vi "Find Multiple by Path Test.vi"() -> ()   [LabVIEW 2017]
uses:
  String Subset.vi
  support/Strip Quotes and Unescape.vi
  Parsing/Parse Full Path or Item Name.vi
  Offset/Find Item Locations by Path.vi
  support/Unescape JSON string.vi
  support/Format JSON Object.vi
  <vilib>/addons/_JKI Toolkits/Caraya/classes/Test/Test.lvclass
  <vilib>/addons/_JKI Toolkits/Caraya/classes/Assert/Assert.lvclass
  JSONtext.lvlib
panel:
  out "Array":string[](array[string])
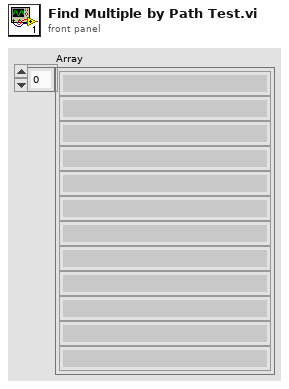
[diagram p1: front panel]
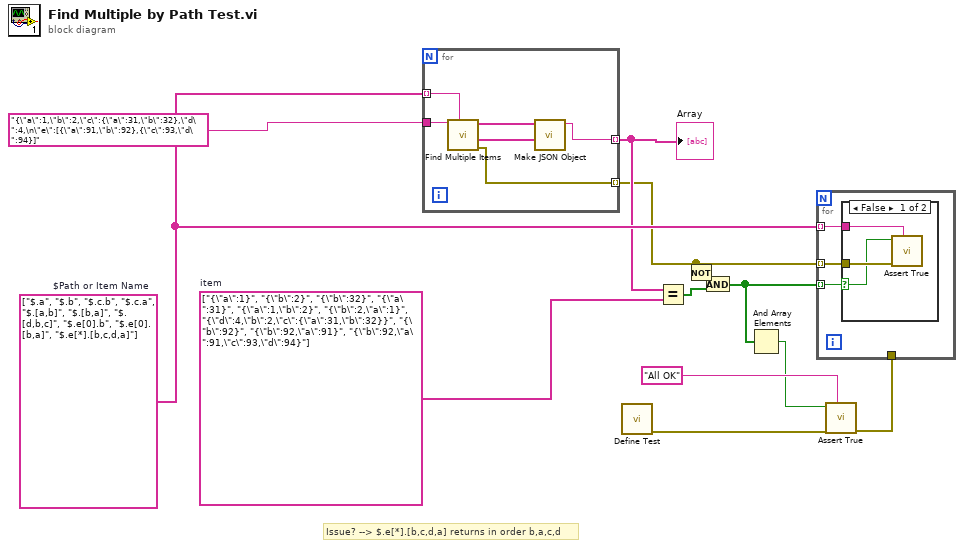
[diagram p0: block diagram]
diagram:
  w1 = string[] ["{\"a\":1}", "{\"b\":2}", "{\"b\":32}", "{\"a\":31}", "{\"a\":1,\"b\":2}", "{\"b\":2,\"a\":1}", "{\"d\":4,\"b\":2,\"c\":{\"a\":31,\"b\":32}}", "{\"b\":92}", "{\"b\":92,\"a\":91}", "{\"b\":92,\"a\":91,\"c\":93,\"d\":94}"]  # item
  w11 = string[] ["$.a", "$.b", "$.c.b", "$.c.a", "$.[a,b]", "$.[b,a]", "$.[d,b,c]", "$.e[0].b", "$.e[0].[b,a]", "$.e[*].[b,c,d,a]"]  # $Path or Item Name
  # "Issue? --> $.e[*].[b,c,d,a] returns in order b,a,c,d"
  n1 = for {
    tunnel: "{\"a\":1,\"b\":2,\"c\":{\"a\":31,\"b\":32},\"d\":4,\n\"e\":[{\"a\":91,\"b\":92},{\"c\":93,\"d\":94}]" -> [w18]
    tunnel: w11 -> [w17] mode=indexing
    tunnel: [w13] -> w8 mode=indexing
    tunnel: [w16] -> w6 mode=indexing
    n2 = call "Find Multiple Items.vi"("$Path or Item Name"=w17, "JSON"=w18) -> ("error out"=w16:errorcluster, "<JSON>"=w15:string[], "Item Names"=w14:string[])  [unwired: 6 in, 1 out]
    n3 = call "Make JSON Object.vi"("JSON Items"=w15, "Item Names"=w14) -> ("<JSON>"=w13:string)  [unwired: 8 in, 1 out]
  }
  "Array" <- w8
  n4 = call <vilib>:"Define Test.vi"() -> ("error out"=w10:errorcluster)  [unwired: 11 in]
  n5 = Equal?(x=w8, y=w1) -> (x = y?=w7:bool[])
  n6 = Not(x=w6) -> (.not. x?=w5:bool[])
  n7 = And(x=w5, y=w7) -> (x .and. y?=w4:bool[])
  n8 = And Array Elements(Boolean array=w4) -> (logical AND=w3:bool)
  n9 = call <vilib>:"Assert True.vi"("Label"="All OK", "error in (no error)"=w10, "True?"=w3) -> ("error out"=w2:errorcluster)  [unwired: 8 in]
  n10 = for {
    tunnel: w11 -> [w21] mode=indexing
    tunnel: w6 -> [w20] mode=indexing
    tunnel: w4 -> [w19] mode=indexing
    tunnel: w2 -> [_]
    n11 = case shown="False" w19 {
      selector: w19 -> [w22 _]
      tunnel: w21 -> [w24 _]
      tunnel: w20 -> [w23 _]
      frame False {
        n12 = call <vilib>:"Assert True.vi"("Label"=w24, "error in (no error)"=w23, "True?"=w22) -> ()  [unwired: 8 in, 1 out]
      }
      frame True {
      }
    }
  }
